vi "AddMessage.vi"(4 "add newline":bool, 5 "message":string, 6 "error in":errorcluster, 9 "RasPi Compiler in":refnum<class "RasPi Compiler.lvclass">) -> (0 "error out":errorcluster, 3 "RasPi Compiler out":refnum<class "RasPi Compiler.lvclass">)   [LabVIEW 2014, in "Raspberry Pi Compatible Compiler for LabVIEW.lvlib" / "RasPi Compiler.lvclass"]
uses:
  RasPi Compiler.lvclass
  RasPi Compiler.lvclass/RasPi Compiler.ctl
  RasPi_Services/MessageBox/MessageBox.lvclass
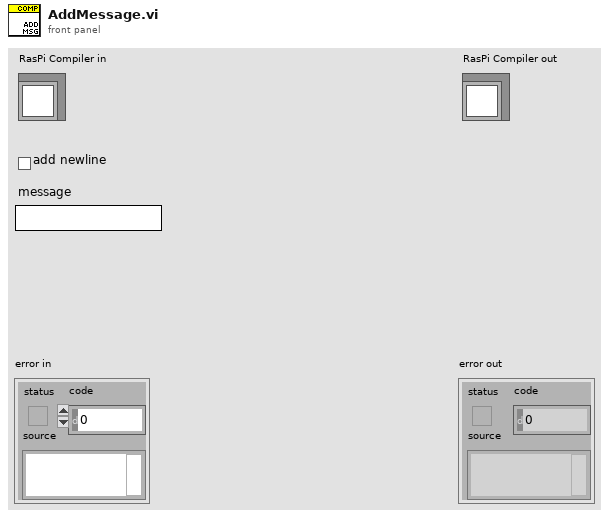
[diagram p1: front panel]
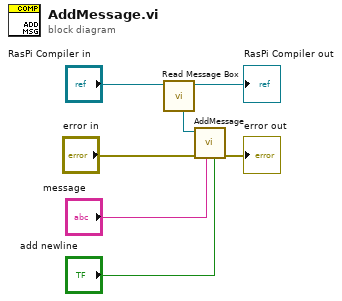
[diagram p0: block diagram]
diagram:
  n1 = call "Read Message Box.vi"("RasPi Compiler in"="RasPi Compiler in") -> ("RasPi Compiler out"=→"RasPi Compiler out":refnum<class "RasPi Compiler.lvclass">, "Message Box"=w5:refnum<class "MessageBox.lvclass">)  [unwired: 7 in]
  n2 = call "AddMessage.vi"("add newline"="add newline", "message"="message", "error in"="error in", "MessageBox in"=w5) -> ("error out"=→"error out":errorcluster)  [unwired: 4 in, 1 out]
